vi "getActorType.vi"(8 "error in":errorcluster, 9 "Actor Type":dbl, 10 "axis in":u8, 11 "connection ID":refnum<k5>) -> (0 "error out":errorcluster, 1 "Actor Type":dbl, 2 "axis out":u8, 3 "connection ID":refnum<k5>)   [LabVIEW 2016]
panel:
  in  "Get Command":string="com.attocube.amc.control.getActorType"
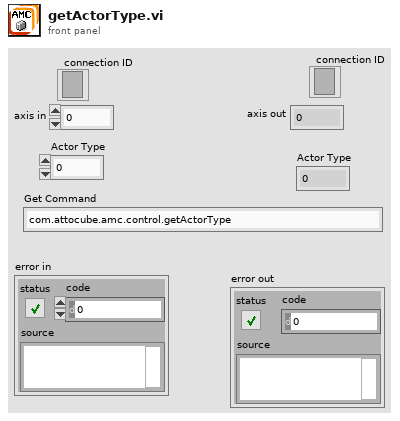
[diagram p1: front panel]
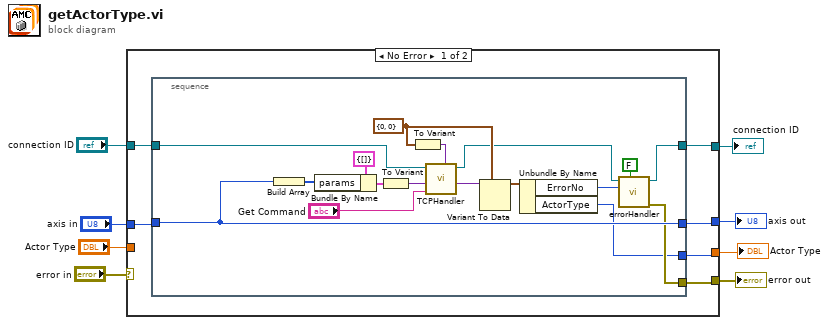
[diagram p0: block diagram]
diagram:
  n1 = case shown="No Error" "error in" {
    selector: "error in" -> [_ w35]
    tunnel: "axis in" -> [w13 w33]
    tunnel: [w9 w35] -> w7
    tunnel: [w11 w33] -> w6
    tunnel: [w10 w32] -> w5
    tunnel: "connection ID" -> [w14 w32]
    tunnel: [w12 w34] -> w3
    tunnel: "Actor Type" -> [_ w34]
    frame No Error {
      n2 = stacked-sequence {
        tunnel: [w15] -> w10
        tunnel: w14 -> [w21]
        tunnel: w13 -> [w23]
        tunnel: [w23] -> w11
        tunnel: [w22] -> w9
        tunnel: [w18] -> w12
        frame #0 {
          w19 = cluster{"ErrorNo":i16, "ActorType":i64} {"ErrorNo"=0, "ActorType"=0} ("input cluster")
          n3 = Build Array(w23) -> (w27:u8[])
          n4 = Bundle By Name(cluster=cluster{"params":i16[]} {"params"=[]} ("input cluster"), "params"=w27) -> (w28:cluster{"params":i16[]})
          n5 = To Variant(anything=w28) -> (Variant=w29:variant)
          n6 = To Variant(anything=w19) -> (Variant=w20:variant)
          n7 = call "TCPHandler.vi"("result Types"=w20, "method"="Get Command", "params"=w29, "connection ID"=w21) -> ("result"=w25:variant, "connection ID"=w16:refnum<k5>)  [unwired: 5 in, 1 out]
          n8 = Variant To Data(type=w19, Variant=w25) -> (data=w30:cluster{"ErrorNo":i16, "ActorType":i64})  [unwired: 1 in, 1 out]
          n9 = Unbundle By Name(w30) -> ("ErrorNo"=w31:i16, "ActorType"=w18:i64)
          n10 = call "errorHandler.vi"("show popup"=FALSE, "error number"=w31, "connection ID"=w16) -> ("error out"=w22:errorcluster, "connection ID"=w15:refnum<k5>)  [unwired: 7 in]
        }
      }
    }
    frame Error {
    }
  }
  "error out" <- w7
  "axis out" <- w6
  "connection ID" <- w5
  "Actor Type" <- w3
